vi "generateSignedGaussians.vi"(6 "timeout (10000)":i32=10000, 8 "error in (no error)":errorcluster, 11 "Parameters":T2) -> (0 "error out":errorcluster, 3 "Response":T1 {"result"."random"."data" format="%#_14g"}, 4 "error data":string[](array[string]))   [LabVIEW 2014, in "Random JSON API.lvlib"]
uses:
  Random JSON API.lvlib
  Type Defs/generateGaussiansRequest.ctl
  Type Defs/generateSignedGaussiansResponse.ctl
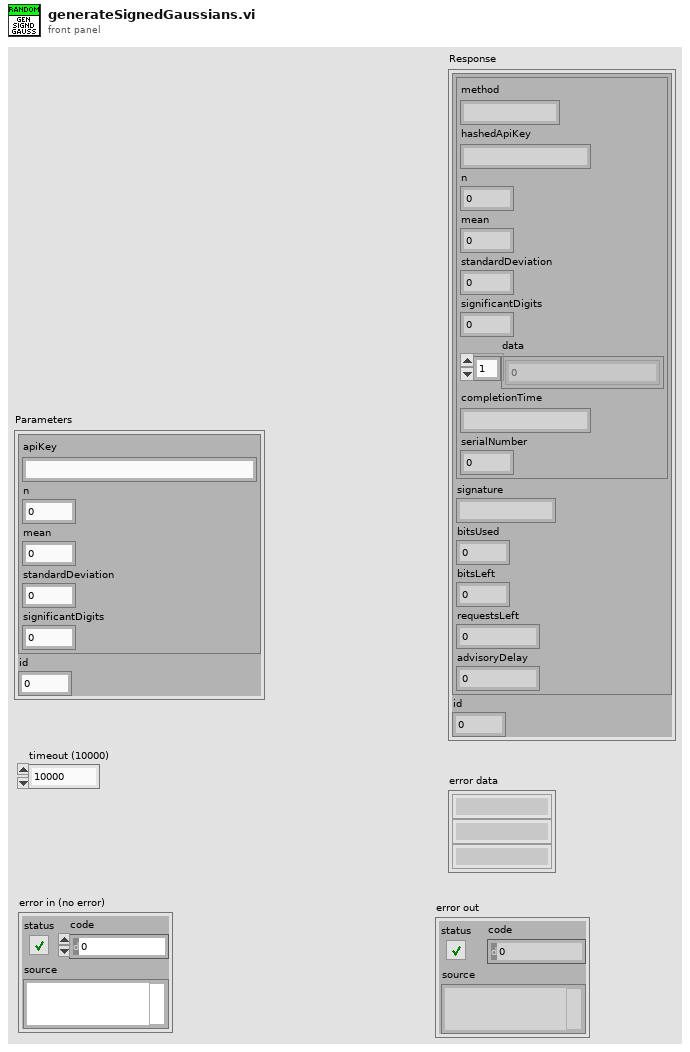
[diagram p1: front panel]
types:
  T1 = typedef "Random JSON API.lvlib/generateSignedGaussiansResponse.ctl" = cluster{"result":cluster{"random":cluster{"method":string, "hashedApiKey":string, "n":i32, "mean":dbl, "standardDeviation":dbl, "significantDigits":i32, "data":dbl[], "completionTime":string, "serialNumber":i32}, "signature":string, "bitsUsed":i32, "bitsLeft":i32, "requestsLeft":i32, "advisoryDelay":i32}, "id":dbl}
  T2 = typedef "Random JSON API.lvlib/generateGaussiansRequest.ctl" = cluster{"params":cluster{"apiKey":string, "n":i32, "mean":dbl, "standardDeviation":dbl, "significantDigits":i32}, "id":dbl}
  T3 = cluster{"apiKey":string, "n":i32, "mean":dbl, "standardDeviation":dbl, "significantDigits":i32}
  T4 = cluster{"jsonrpc":string, "method":string, "params":cluster{"apiKey":string, "n":i32, "mean":dbl, "standardDeviation":dbl, "significantDigits":i32}, "id":dbl}
  T5 = cluster{"result cluster":cluster{"completionTime":string, "bitsUsed":i32, "bitsLeft":i32, "requestsLeft":i32, "advisoryDelay":i32}, "method":string, "hashedApiKey":string, "n":i32, "serialNumber":i32, "signature":string}
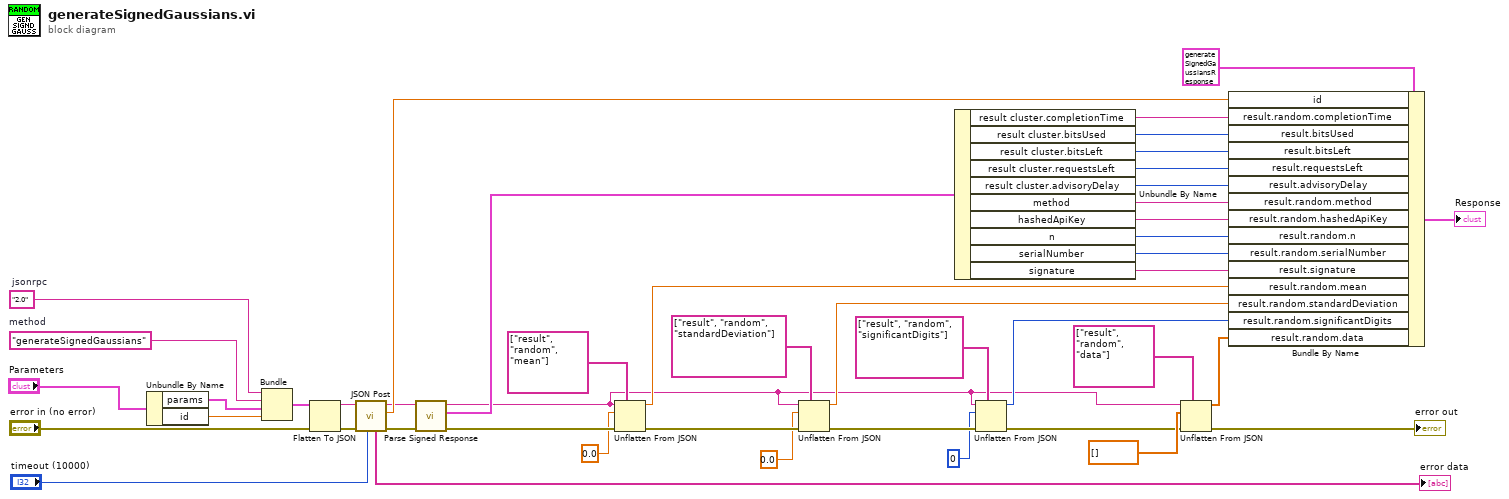
[diagram p0: block diagram]
diagram:
  w36 = "2.0"  # jsonrpc
  w38 = "generateSignedGaussians"  # method
  n1 = Unbundle By Name("Parameters") -> ("params"=w35:T3, "id"=w37:dbl)
  n2 = Bundle("jsonrpc"=w36, "method"=w38, "params"=w35, "id"=w37) -> (w31:T4)  [unwired: 1 in]
  n3 = Flatten To JSON(anything=w31, error in (no error)="error in (no error)") -> (JSON string=w32:string, 11:w33:errorcluster)  [unwired: 1 in]
  n4 = call "JSON Post.vi"("timeout (10000)"="timeout (10000)", "error in (no error)"=w33, "Request JSON String"=w32) -> ("error out"=w44:errorcluster, "id"=w28:dbl, "Response JSON String"=w27:string, "error data"=→"error data":string[])  [unwired: 5 in]
  n5 = call "Parse Signed Response.vi"("error in (no error)"=w44, "body in"=w27) -> ("error out"=w11:errorcluster, "signed result cluster"=w26:T5, "body out"=w1:string)  [unwired: 7 in]
  n6 = Unflatten From JSON(path=string[] ["result", "random", "mean"], JSON string=w1, type and defaults=0.0, error in (no error)=w11) -> (value=w5:dbl, error out=w10:errorcluster)  [unwired: 3 in]
  n7 = Unflatten From JSON(path=string[] ["result", "random", "standardDeviation"], JSON string=w1, type and defaults=0.0, error in (no error)=w10) -> (value=w6:dbl, error out=w9:errorcluster)  [unwired: 3 in]
  n8 = Unbundle By Name(w26) -> ("result cluster.completionTime"=w43:string, "result cluster.bitsUsed"=w42:i32, "result cluster.bitsLeft"=w41:i32, "result cluster.requestsLeft"=w40:i32, "result cluster.advisoryDelay"=w39:i32, "method"=w21:string, "hashedApiKey"=w20:string, "n"=w19:i32, "serialNumber"=w18:i32, "signature"=w17:string)
  n9 = Unflatten From JSON(path=string[] ["result", "random", "significantDigits"], JSON string=w1, type and defaults=0, error in (no error)=w9) -> (value=w7:i32, error out=w8:errorcluster)  [unwired: 3 in]
  n10 = Unflatten From JSON(path=string[] ["result", "random", "data"], JSON string=w1, type and defaults=dbl[] [], error in (no error)=w8) -> (value=w16:dbl[], error out=→"error out":errorcluster)  [unwired: 3 in]
  n11 = Bundle By Name(cluster=T1 {"result"={"random"={"method"="", "hashedApiKey"="", "n"=0, "mean"=0.0, "standardDeviation"=0.0, "significantDigits"=0, "data"=[], "completionTime"="", "serialNumber"=0}, "signature"="", "bitsUsed"=0, "bitsLeft"=0, "requestsLeft"=0, "advisoryDelay"=0}, "id"=0.0} ("Response"), "id"=w28, "result.random.completionTime"=w43, "result.bitsUsed"=w42, "result.bitsLeft"=w41, "result.requestsLeft"=w40, "result.advisoryDelay"=w39, "result.random.method"=w21, "result.random.hashedApiKey"=w20, "result.random.n"=w19, "result.random.serialNumber"=w18, "result.signature"=w17, "result.random.mean"=w5, "result.random.standardDeviation"=w6, "result.random.significantDigits"=w7, "result.random.data"=w16) -> (→"Response":T1)
